vi "Configure Power Analysis (Harmonics).vi"(5 "User Defined Real Power (70 W)":dbl=70.0, 7 "Enable User Defined Power (F: Disable)":bool, 8 "error in (no error)":errorcluster, 9 "Standard (0: IEC 61000- 3- 2 Class A)":i32(ring) items=["IEC 61000- 3- 2 Class A", "IEC 61000- 3- 2 Class B", "IEC 61000- 3- 2 Class C", "IEC 61000- 3- 2 Class D"], 10 "Line Frequency (0: 50 Hz)":i32(ring) items=["50 Hz", "60 Hz", "400 Hz"], 11 "VISA resource name":refnum<visa-resource-name>) -> (0 "error out":errorcluster, 3 "VISA resource name out":refnum<visa-resource-name>)   [LabVIEW 2023, in "Keysight-DSQx3014T.lvlib"]
doc: "Applies the current harmonics analysis.\n\n<B>Note(s):</B>\nSwitching power supplies draw a range of harmonics from the AC mains.\n\nStandard limits are set for these harmonics because these harmonics can travel back to the supply grid and cause problems with other devices on the grid.\n\nUse the Current Harmonics analysis to test a switching power supply's current harmonics to pre-compliance standard of IEC61000- 3- 2 (Class A, B, C, or D). The analysis presents up to 40 harmonics.\n\nUse <B>Read Measurement (Harmonics Power Analysis).vi</B> to read the result of this power analysis."
uses:
  Keysight-DSQx3014T.lvlib
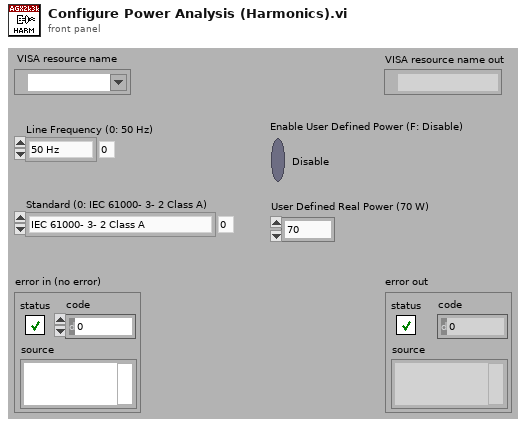
[diagram p1: front panel]
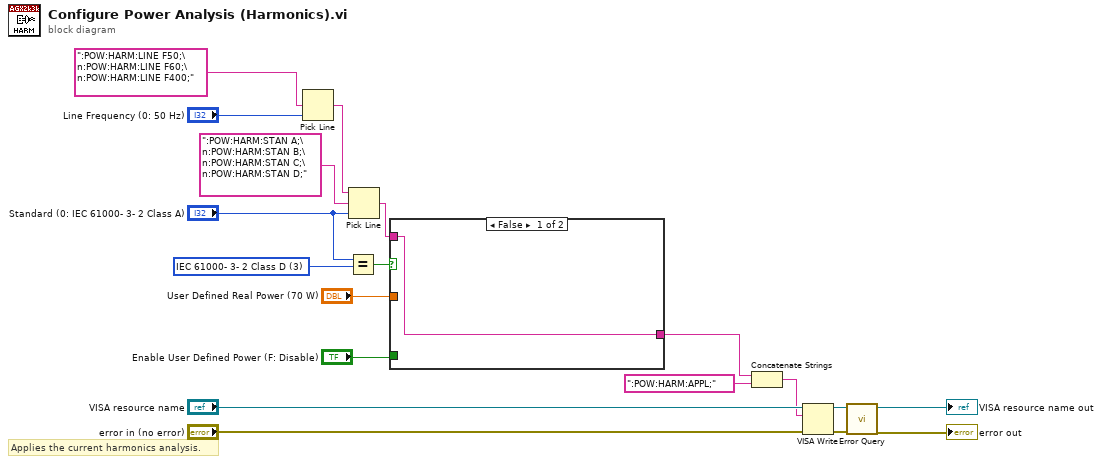
[diagram p0: block diagram]
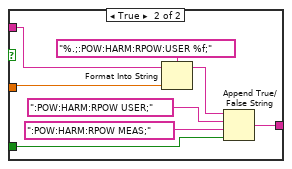
[diagram p2: hidden frame]
diagram:
  w2 = 3 items=["IEC 61000- 3- 2 Class A", "IEC 61000- 3- 2 Class B", "IEC 61000- 3- 2 Class C", "IEC 61000- 3- 2 Class D"] ("Standard (0: IEC 61000- 3- 2 Class A)")
  # "Applies the current harmonics analysis."
  n1 = Pick Line(multi-line string=":POW:HARM:LINE F50;\n:POW:HARM:LINE F60;\n:POW:HARM:LINE F400;", line index="Line Frequency (0: 50 Hz)") -> (output string=w16:string)  [unwired: 1 out]
  n2 = Equal?(x="Standard (0: IEC 61000- 3- 2 Class A)", y=w2) -> (x = y?=w1:bool)
  n3 = Pick Line(string ("")=w16, multi-line string=":POW:HARM:STAN A;\n:POW:HARM:STAN B;\n:POW:HARM:STAN C;\n:POW:HARM:STAN D;", line index="Standard (0: IEC 61000- 3- 2 Class A)") -> (output string=w6:string)
  n4 = case shown="False" w1 {
    tunnel: "User Defined Real Power (70 W)" -> [_ w27]
    tunnel: w6 -> [w20 w26]
    tunnel: [w20 w24] -> w5
    tunnel: "Enable User Defined Power (F: Disable)" -> [_ w23]
    frame False {
    }
    frame True {
      n5 = Format Into String(format string="%.;:POW:HARM:RPOW:USER %f;", initial string=w26, w27) -> (resulting string=w25:string)  [unwired: 1 in, 1 out]
      n6 = Append True/False String(1:w23, 2:":POW:HARM:RPOW MEAS;" ("true string"), 3:":POW:HARM:RPOW USER;" ("false string"), 4:w25) -> (0:w24:string)
    }
  }
  n7 = Concatenate Strings(w5, ":POW:HARM:APPL;") -> (w8:string)
  n8 = VISA Write(VISA resource name="VISA resource name", write buffer=w8, error in (no error)="error in (no error)") -> (VISA resource name out=w13:refnum<visa-resource-name>, error out=w12:errorcluster)  [unwired: 1 out]
  n9 = call "Error Query.vi"("error in (no error)"=w12, "VISA resource name"=w13) -> ("error out"=→"error out":errorcluster, "VISA resource name out"=→"VISA resource name out":refnum<visa-resource-name>)  [unwired: 8 out]
